vi "RSZVB Set ALC Port Start Offset.vi"(7 "Start Offset (0.0)":dbl format="%^.3e", 8 "error in (no error)":errorcluster {"code" format="%.0x"}, 9 "Port (1)":i32=1, 10 "Channel (1)":i32=1, 11 "VISA session":refnum<visa-resource-name>) -> (0 "error out":errorcluster {"code" format="%.0x"}, 3 "dup VISA session":refnum<visa-resource-name>)   [LabVIEW 2011]
doc: "Defines the signal level before the ALC loop is started (Start Value > Offset in ALC Config dialog) for port <Pt> in channel <Ch>. \n\nRemote-control command(s):\nSOURce<Ch>:POWer<Pt>:ALC:SOFFset"
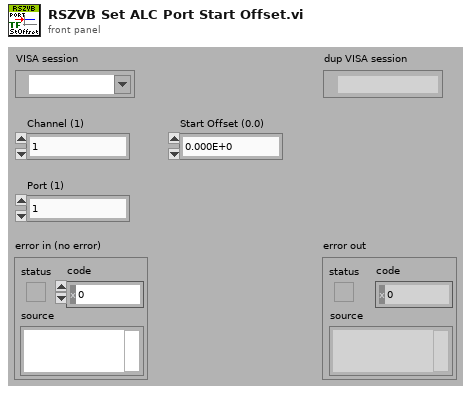
[diagram p1: front panel]
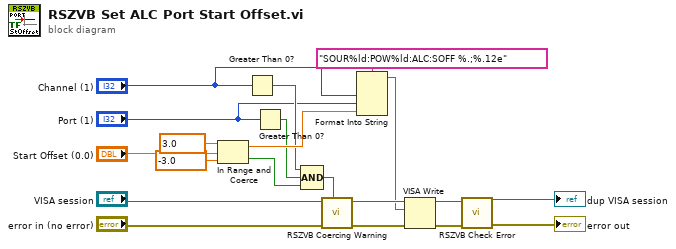
[diagram p0: block diagram]
diagram:
  n1 = In Range and Coerce(upper limit=3.0, x="Start Offset (0.0)", lower limit=-3.0) -> (coerced(x)=w12:dbl, In Range?=w11:bool)
  n2 = Greater Than 0?(x="Channel (1)") -> (x > 0?=w9:bool)
  n3 = Greater Than 0?(x="Port (1)") -> (x > 0?=w10:bool)
  n4 = Compound Arithmetic op=AND(w9, w10, w11) -> (w8:bool)
  n5 = call "RSZVB Coercing Warning.vi"("In Range?"=w8, "error in (no error)"="error in (no error)", "VISA session"="VISA session") -> ("error out"=w18:errorcluster, "dup VISA session"=w19:refnum<visa-resource-name>)  [unwired: 7 in]
  n6 = Format Into String(format string="SOUR%ld:POW%ld:ALC:SOFF %.;%.12e", "Channel (1)", "Port (1)", w12) -> (resulting string=w15:string)  [unwired: 2 in, 1 out]
  n7 = VISA Write(VISA resource name=w19, write buffer=w15, error in (no error)=w18) -> (VISA resource name out=w16:refnum<visa-resource-name>, error out=w17:errorcluster)  [unwired: 1 out]
  n8 = call "RSZVB Check Error.vi"("error in (no error)"=w17, "VISA session"=w16) -> ("error out"=→"error out":errorcluster, "dup VISA session"=→"dup VISA session":refnum<visa-resource-name>)  [unwired: 8 in]
